vi "ShiftRegisterMarcoGonzalez.vi"() -> ()   [LabVIEW 2012]
panel:
  out "Bottom Final":dbl
  out "Top Final":dbl
  out "Bottom Second":dbl
  out "Bottom New":dbl
  out "Top Second":dbl
  out "Top New":dbl
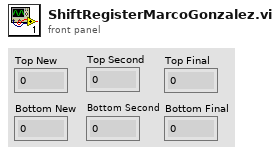
[diagram p1: front panel]
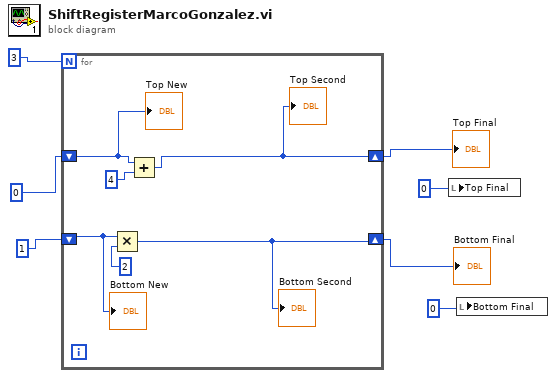
[diagram p0: block diagram]
diagram:
  n1 = for {
    N: 3 -> [_]
    shift-right: [w11] -> w4
    shift-left: 0 -> [w10]
    shift-right: [w8] -> w3
    shift-left: 1 -> [w9]
    n2 = Multiply(x=w9, y=2) -> (x*y=w8:i32)
    "Bottom Second" <- w8
    n3 = Add(x=w10, y=4) -> (x+y=w11:i32)
    "Top Second" <- w11
    "Top New" <- w10
    "Bottom New" <- w9
  }
  "Top Final" <- w4
  "Bottom Final" <- w3
  n4 = local write "Top Final"(0) -> ()
  n5 = local write "Bottom Final"(0) -> ()
